vi "assignName.vi"(6 "recurse":bool=TRUE, 8 "error in (no error)":errorcluster, 10 "subNode in":refnum<data-value>, 11 "superNode in":refnum<class "xceDataNode.lvclass">) -> (0 "error out":errorcluster, 2 "subNode out":refnum<data-value>, 3 "superNode out":refnum<class "xceDataNode.lvclass">)   [LabVIEW 2013, in "xceDataNode.lvclass"]
doc: "Assigns an original name to the xceDataNode based on the names of the other xceDataNodes that have the same supernode."
uses:
  xceDataNode.lvclass
  xceNode/xceNode.lvclass
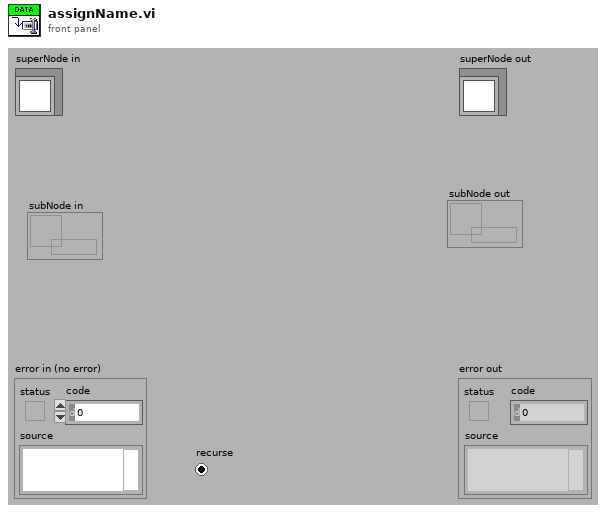
[diagram p1: front panel]
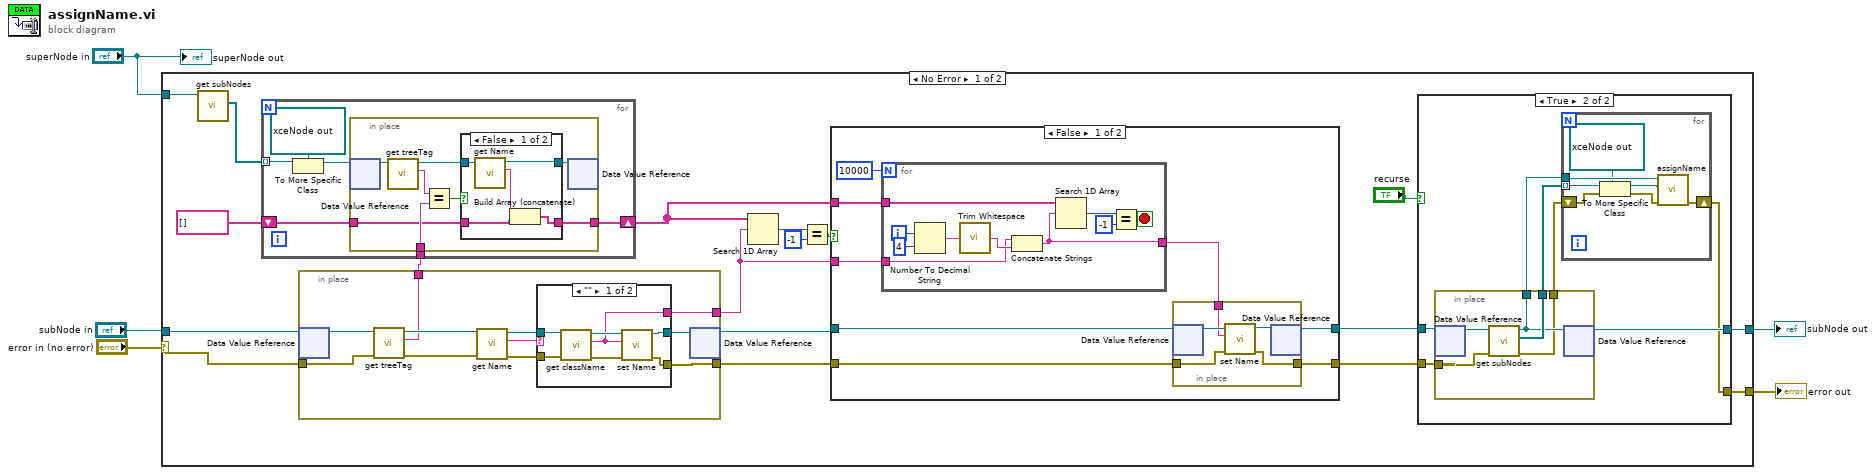
[diagram p0: block diagram]
diagram:
  n1 = case shown="No Error" "error in (no error)" {
    selector: "error in (no error)" -> [w9 w113]
    tunnel: [w14 w113] -> w4
    tunnel: "superNode in" -> [w23 _]
    tunnel: "subNode in" -> [w10 w112]
    tunnel: [w15 w112] -> w1
    frame No Error {
      n2 = call "get subNodes.vi"("xceNode in"=w23) -> ("subNodes[]*"=w22:refnum<data-value>[])  [unwired: 8 in, 2 out]
      n3 = in-place {
        in-place-border: [w76] -> w11
        in-place-border: w9 -> [w72]
        in-place-border: [w75] -> w13
        in-place-border: [w70] -> w7
        n4 = in-place-dvr #1(w10) -> (w74:refnum<class "xceDataNode.lvclass">)  [unwired: 1 out]
        n5 = call "get treeTag.vi"("error in (no error)"=w72, "xceNode in"=w74) -> ("error out"=w71:errorcluster, "treeTag"=w70:string, "xceNode out"=w73:refnum<class "xceDataNode.lvclass">)  [unwired: 7 in]
        n6 = call "get Name.vi"("error in (no error)"=w71, "xceDataNode in"=w73) -> ("error out"=w78:errorcluster, "Name"=w80:string, "xceDataNode out"=w79:refnum<class "xceDataNode.lvclass">)  [unwired: 7 in]
        n7 = case shown="\"\"" w80 {
          selector: w80 -> [_ w89]
          tunnel: w79 -> [w87 w90]
          tunnel: w78 -> [w86 w88]
          tunnel: [w84 w90] -> w77
          tunnel: [w83 w89] -> w76
          tunnel: [w81 w88] -> w75
          frame "" {
            n8 = call "get className.vi"("error in (no error)"=w86, "xceNode in"=w87) -> ("error out"=w82:errorcluster, "Class name"=w83:string, "xceNode out"=w85:refnum<class "xceDataNode.lvclass">)  [unwired: 7 in]
            n9 = call "set Name.vi"("error in (no error)"=w82, "Name"=w83, "xceDataNode in"=w85) -> ("error out"=w81:errorcluster, "xceDataNode out"=w84:refnum<class "xceDataNode.lvclass">)  [unwired: 7 in]
          }
          frame Default {
          }
        }
        n10 = in-place-dvr #1(w77) -> (w17:refnum<data-value>)  [unwired: 1 out]
      }
      n11 = for {
        tunnel: w22 -> [w96] mode=indexing
        tunnel: w7 -> [w93]
        shift-right: [w91] -> w18
        shift-left: string[] [] -> [w92]
        n12 = To More Specific Class(target class=refnum<data-value> refnum ("data value reference"), reference=w96) -> (specific class reference=w95:refnum<data-value>)  [unwired: 1 in, 1 out]
        n13 = in-place {
          in-place-border: w93 -> [w102]
          in-place-border: w92 -> [w98]
          in-place-border: [w97] -> w91
          n14 = in-place-dvr #2(w95) -> (w104:refnum<class "xceDataNode.lvclass">)  [unwired: 1 out]
          n15 = call "get treeTag.vi"("xceNode in"=w104) -> ("treeTag"=w103:string, "xceNode out"=w100:refnum<class "xceDataNode.lvclass">)  [unwired: 8 in, 1 out]
          n16 = Equal?(x=w103, y=w102) -> (x = y?=w101:bool)
          n17 = case shown="False" w101 {
            tunnel: w100 -> [w109 w111]
            tunnel: [w108 w111] -> w99
            tunnel: w98 -> [w106 w110]
            tunnel: [w105 w110] -> w97
            frame False {
              n18 = call "get Name.vi"("xceDataNode in"=w109) -> ("Name"=w107:string, "xceDataNode out"=w108:refnum<class "xceDataNode.lvclass">)  [unwired: 8 in, 1 out]
              n19 = Build Array (concatenate)(w107, w106) -> (w105:string[])
            }
            frame True {
            }
          }
          n20 = in-place-dvr #2(w99) -> ()  [unwired: 2 out]
        }
      }
      n21 = Search 1D Array(1D array=w18, element=w11) -> (index of element=w21:i32)  [unwired: 1 in]
      n22 = Equal?(x=w21, y=-1) -> (x = y?=w19:bool)
      n23 = case shown="False" w19 {
        tunnel: w18 -> [w50 _]
        tunnel: w17 -> [w49 w69]
        tunnel: [w48 w69] -> w16
        tunnel: w13 -> [w46 w68]
        tunnel: [w45 w68] -> w12
        tunnel: w11 -> [w51 _]
        frame False {
          n24 = for {
            N: 10000 -> [_]
            tunnel: w51 -> [w58]
            tunnel: w50 -> [w64]
            tunnel: [w60] -> w47
            i -> [w67]
            stop <- w61 stop-if-true
            n25 = Number To Decimal String(number=w67, width (-)=i16 4) -> (decimal integer string=w65:string)
            n26 = call <vilib>:"Trim Whitespace.vi"("string"=w65) -> ("trimmed string"=w59:string)  [unwired: 1 in]
            n27 = Concatenate Strings(w58, w59) -> (w60:string)
            n28 = Search 1D Array(1D array=w64, element=w60) -> (index of element=w63:i32)  [unwired: 1 in]
            n29 = Equal?(x=w63, y=-1) -> (x = y?=w61:bool)
          }
          n30 = in-place {
            in-place-border: w47 -> [w56]
            in-place-border: w46 -> [w55]
            in-place-border: [w54] -> w45
            n31 = in-place-dvr #3(w49) -> (w57:refnum<class "xceDataNode.lvclass">)  [unwired: 1 out]
            n32 = call "set Name.vi"("error in (no error)"=w55, "Name"=w56, "xceDataNode in"=w57) -> ("error out"=w54:errorcluster, "xceDataNode out"=w53:refnum<class "xceDataNode.lvclass">)  [unwired: 7 in]
            n33 = in-place-dvr #3(w53) -> (w48:refnum<data-value>)  [unwired: 1 out]
          }
        }
        frame True {
        }
      }
      n34 = case shown="True" "recurse" {
        tunnel: w16 -> [w25 w32]
        tunnel: [w25 w29] -> w15
        tunnel: [w24 w27] -> w14
        tunnel: w12 -> [w24 w26]
        frame False {
        }
        frame True {
          n35 = in-place {
            in-place-border: [w43] -> w31
            in-place-border: [w42] -> w30
            in-place-border: [w41] -> w28
            in-place-border: w26 -> [w40]
            n36 = in-place-dvr #4(w32) -> (w44:refnum<class "xceDataNode.lvclass">)  [unwired: 1 out]
            n37 = call "get subNodes.vi"("error in (no error)"=w40, "xceNode in"=w44) -> ("error out"=w41:errorcluster, "subNodes[]*"=w43:refnum<data-value>[], "xceNode out"=w42:refnum<class "xceDataNode.lvclass">)  [unwired: 7 in]
            n38 = in-place-dvr #4(w42) -> (w29:refnum<data-value>)  [unwired: 1 out]
          }
          n39 = for {
            tunnel: w31 -> [w39] mode=indexing
            tunnel: w30 -> [w38]
            shift-right: [w36] -> w27
            shift-left: w28 -> [w35]
            n40 = To More Specific Class(target class=refnum<data-value> refnum ("subNode in"), reference=w39, error in=w35) -> (specific class reference=w34:refnum<data-value>, error out=w37:errorcluster)
            n41 = call "assignName.vi"("error in (no error)"=w37, "subNode in"=w34, "superNode in"=w38) -> ("error out"=w36:errorcluster)  [unwired: 6 in, 2 out]
          }
        }
      }
    }
    frame Error {
    }
  }
  "error out" <- w4
  "subNode out" <- w1
  "superNode out" <- "superNode in"
